vi "Write All Elements GUI.vi"(8 "error in (no error)":errorcluster, 10 "Temperature params.":T1={"Temperature field"=FALSE, "Ratio correction factor"=1.0, "Temperature value"=FALSE, "Y-coord."=0.0, "X-coord."=0.0, "Averaging center"=enum."Fixed coordinates (mm)", "Averaging shape"=enum."Point", "Minor axis"=0.0, "Major axis"=0.0} {"Major axis" min=0.0; "Minor axis" min=0.0; "Ratio correction factor" min=0.0 step=0.0001 format="%#.4g"}, 11 "Temp params in":refnum<class "CV-Temperature.lvclass">) -> (0 "error out":errorcluster, 3 "Temp params out":refnum<class "CV-Temperature.lvclass">)   [LabVIEW 2013, in "CameraVision.lvlib" / "CV-Temperature.lvclass"]
uses:
  CV-Temperature.lvclass
  Temperature-parameters-gui.ctl
  CV-Temperature.lvclass/CV-Temperature.ctl
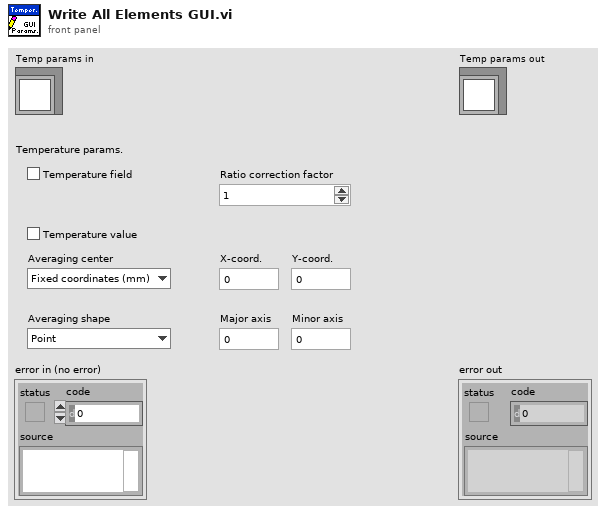
[diagram p1: front panel]
types:
  T1 = typedef "CameraVision.lvlib/CV-Temperature.lvclass/Temperature-parameters-gui.ctl" = cluster{"Temperature field":bool, "Ratio correction factor":dbl, "Temperature value":bool, "Y-coord.":dbl, "X-coord.":dbl, "Averaging center":enum16{"Fixed coordinates (pixel)", "Fixed coordinates (mm)", "Melt-pool center"}, "Averaging shape":enum16{"Point", "Circle", "Ellipse"}, "Minor axis":dbl, "Major axis":dbl}
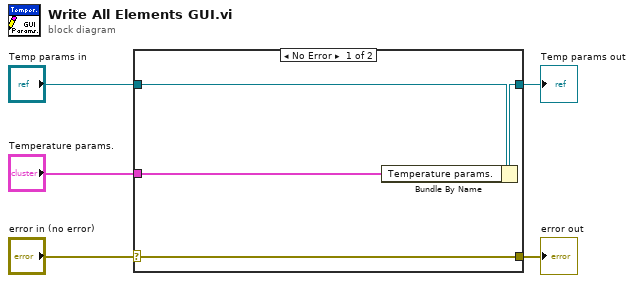
[diagram p0: block diagram]
diagram:
  n1 = case shown="No Error" "error in (no error)" {
    selector: "error in (no error)" -> [w9 w10]
    tunnel: [w9 w10] -> w4
    tunnel: [w7 w11] -> w2
    tunnel: "Temp params in" -> [w8 w11]
    tunnel: "Temperature params." -> [w6 _]
    frame No Error {
      n2 = Bundle By Name(cluster=w8, "Temperature params."=w6) -> (w7:refnum<class "CV-Temperature.lvclass">)
    }
    frame Error {
    }
  }
  "error out" <- w4
  "Temp params out" <- w2
